vi "Tabellen ziehen.vi"(6 "Aktion":T1, 9 "Angehängtes Array":refnum<vi>[](array[refnum]), 10 "Tabelle (Eingang)":refnum<vi>[](array[refnum]), 11 "Konfigurierte Liste Status":refnum<vi>[](array[refnum])) -> ()   [LabVIEW 2020, in "CAN Konfig.lvlib"]
uses:
  Aktion Tabellen ziehen.ctl
  CAN Konfig.lvlib
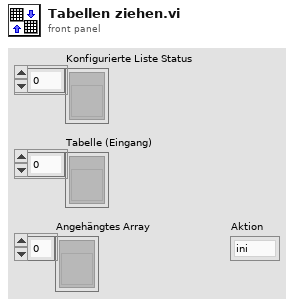
[diagram p1: front panel]
types:
  T1 = typedef "CAN Konfig.lvlib/Aktion Tabellen ziehen.ctl" = enum16{"ini", "prüfen"}
  T2 = enum32{"Optionsauswahl 1", "Optionsauswahl 2", "Optionsauswahl 3"}
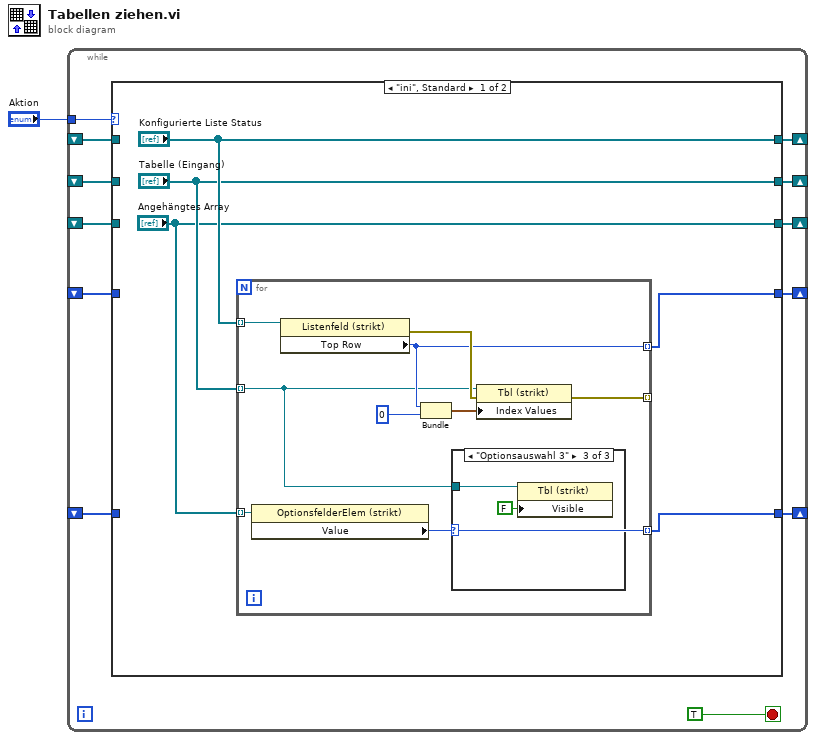
[diagram p0: block diagram]
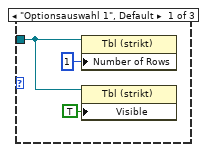
[diagram p2: hidden frame]
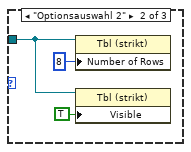
[diagram p3: hidden frame]
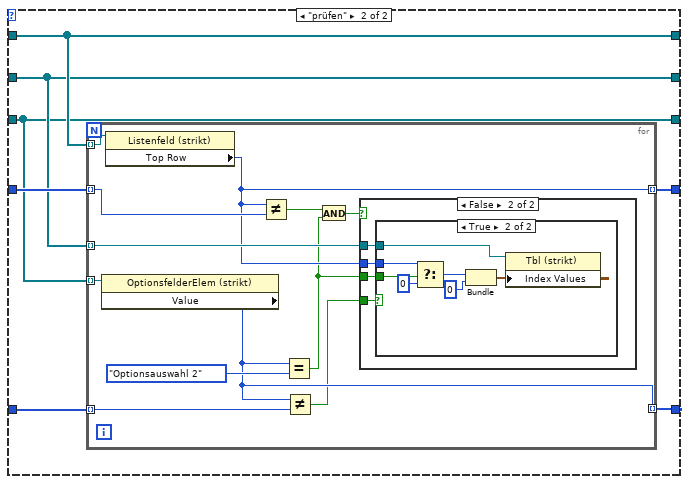
[diagram p4: hidden frame]
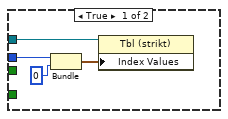
[diagram p5: hidden frame]
diagram:
  n1 = while {
    shift-right: [w13] -> _
    shift-left: _ -> [w11]
    shift-right: [w12] -> _
    shift-left: _ -> [w10]
    tunnel: "Aktion" -> [w9]
    shift-right: [w8] -> _
    shift-left: _ -> [w7]
    shift-right: [w5] -> _
    shift-left: _ -> [w4]
    shift-right: [w3] -> _
    shift-left: _ -> [w2]
    stop <- TRUE stop-if-true
    n2 = case shown="\"ini\", Standard" w9 {
      tunnel: ["Konfigurierte Liste Status" w40] -> w13
      tunnel: ["Tabelle (Eingang)" w39] -> w12
      tunnel: w11 -> [_ w40]
      tunnel: w10 -> [_ w39]
      tunnel: [w16 w42] -> w8
      tunnel: w7 -> [_ w41]
      tunnel: ["Angehängtes Array" w38] -> w5
      tunnel: w4 -> [_ w38]
      tunnel: [w14 w37] -> w3
      tunnel: w2 -> [_ w36]
      frame "ini", Default {
        n3 = for {
          tunnel: "Konfigurierte Liste Status" -> [w25] mode=indexing
          tunnel: "Tabelle (Eingang)" -> [w20] mode=indexing
          tunnel: [w23] -> _ mode=indexing
          tunnel: [w22] -> w16 mode=indexing
          tunnel: "Angehängtes Array" -> [w21] mode=indexing
          tunnel: [w19] -> w14 mode=indexing
          n4 = property class="OptionsfelderElem (strikt)"(reference=w21) -> ("Value"=w19:T2)  [unwired: 1 in, 2 out]
          n5 = property class="Listenfeld (strikt)"(reference=w25) -> (error out=w24:errorcluster, "Top Row"=w22:i32)  [unwired: 1 in, 1 out]
          n6 = Bundle("Top Row"=w22, "Erste Zeile"=0) -> (w27:cluster{"Top Row":i32, "Erste Zeile":i32})  [unwired: 1 in]
          n7 = case shown="\"Optionsauswahl 3\"" w19 {
            tunnel: w20 -> [w28 w31 w34]
            frame "Optionsauswahl 1", Default {
              n8 = property on="Eigenschaftsknoten" class="Tbl (strikt)"(reference=w28, "Number of Rows"=u32 1 ("Zeilenanzahl")) -> ()  [unwired: 1 in, 2 out]
              n9 = property on="Eigenschaftsknoten" class="Tbl (strikt)"(reference=w28, "Visible"=TRUE ("Sichtbar")) -> ()  [unwired: 1 in, 2 out]
            }
            frame "Optionsauswahl 2" {
              n10 = property on="Eigenschaftsknoten" class="Tbl (strikt)"(reference=w31, "Number of Rows"=u32 8 ("Zeilenanzahl")) -> ()  [unwired: 1 in, 2 out]
              n11 = property on="Eigenschaftsknoten" class="Tbl (strikt)"(reference=w31, "Visible"=TRUE ("Sichtbar")) -> ()  [unwired: 1 in, 2 out]
            }
            frame "Optionsauswahl 3" {
              n12 = property on="Eigenschaftsknoten" class="Tbl (strikt)"(reference=w34, "Visible"=FALSE ("Sichtbar")) -> ()  [unwired: 1 in, 2 out]
            }
          }
          n13 = property class="Tbl (strikt)"(reference=w20, error in=w24, "Index Values"=w27) -> (error out=w23:errorcluster)  [unwired: 1 out]
        }
      }
      frame "prüfen" {
        n14 = for {
          tunnel: w40 -> [w54] mode=indexing
          tunnel: [w51] -> w42 mode=indexing
          tunnel: w41 -> [w53] mode=indexing
          tunnel: w39 -> [w52] mode=indexing
          tunnel: w38 -> [w49] mode=indexing
          tunnel: [w46] -> w37 mode=indexing
          tunnel: w36 -> [w45] mode=indexing
          n15 = property class="OptionsfelderElem (strikt)"(reference=w49) -> ("Value"=w46:T2)  [unwired: 1 in, 2 out]
          n16 = property class="Listenfeld (strikt)"(reference=w54) -> ("Top Row"=w51:i32)  [unwired: 1 in, 2 out]
          n17 = Not Equal?(x=w51, y=w53) -> (x != y?=w50:bool)
          n18 = Equal?(x=w46, y=T2."Optionsauswahl 2") -> (x = y?=w43:bool)
          n19 = Not Equal?(x=w46, y=w45) -> (x != y?=w44:bool)
          n20 = And(x=w50, y=w43) -> (x .and. y?=w47:bool)
          n21 = case shown="False" w47 {
            tunnel: w52 -> [w56 w62]
            tunnel: w51 -> [w55 w59]
            tunnel: w44 -> [_ w61]
            tunnel: w43 -> [_ w60]
            frame True {
              n22 = Bundle("Top Row"=w55, "Erste Zeile"=0) -> (w58:cluster{"Top Row":i32, "Erste Zeile":i32})  [unwired: 1 in]
              n23 = property class="Tbl (strikt)"(reference=w56, "Index Values"=w58) -> ()  [unwired: 1 in, 2 out]
            }
            frame False {
              n24 = case shown="True" w61 {
                tunnel: w62 -> [_ w68]
                tunnel: w60 -> [_ w64]
                tunnel: w59 -> [_ w63]
                frame False {
                }
                frame True {
                  n25 = Select(t=w63, s=w64, f=0 ("Erste Zeile")) -> (s? t:f=w66:i32)
                  n26 = Bundle("Erste Zeile"=w66, "Erste Zeile"=0) -> (w69:cluster{"Erste Zeile":i32, "Erste Zeile":i32})  [unwired: 1 in]
                  n27 = property class="Tbl (strikt)"(reference=w68, "Index Values"=w69) -> ()  [unwired: 1 in, 2 out]
                }
              }
            }
          }
        }
      }
    }
  }
